vi "DES.vi"(8 "error in":errorcluster, 9 "keyStr":string="luxshare", 10 "sourceData":string="Figoba", 11 "操作":enum16{"DES_Encrypt", "DES_Decrypt"}(ring)) -> (0 "error out":errorcluster, 3 "加密后字符串":string)   [LabVIEW 2011]
uses:
  Data/DES_string.dll
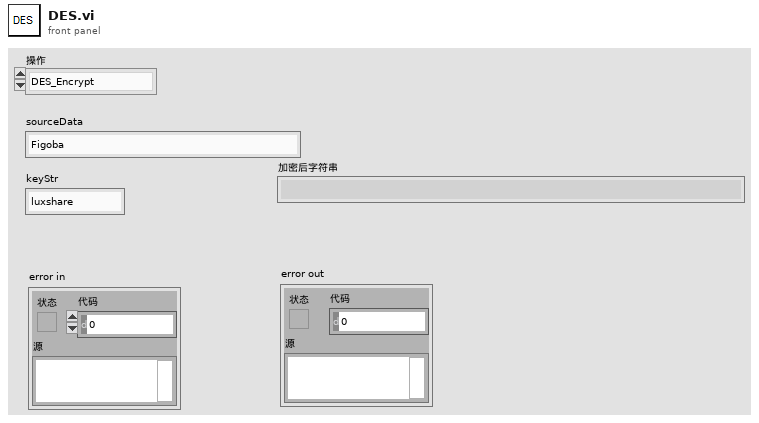
[diagram p1: front panel]
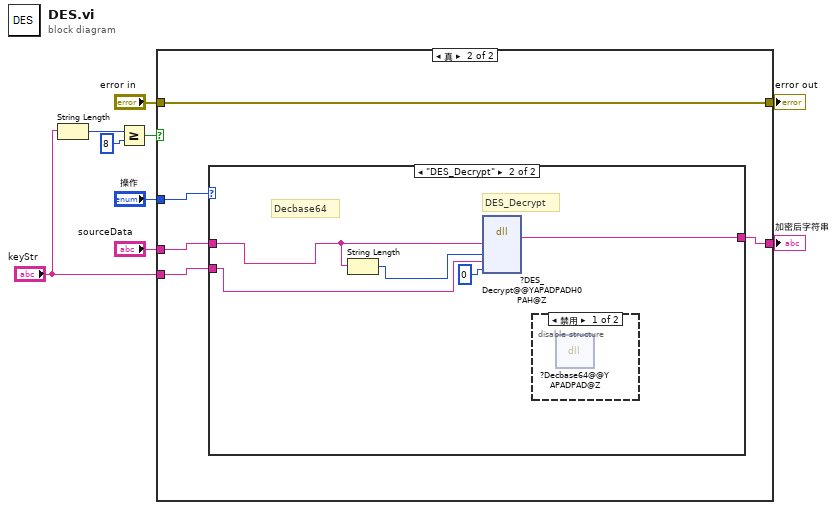
[diagram p0: block diagram]
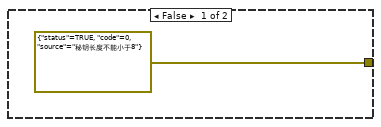
[diagram p2: hidden frame]
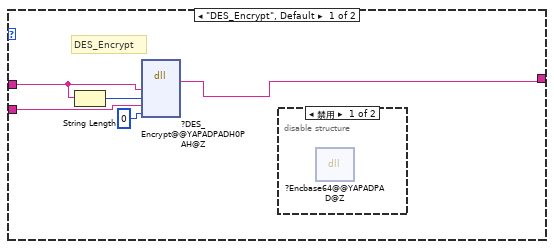
[diagram p3: hidden frame]
diagram:
  n1 = String Length(string="keyStr") -> (length=w9:i32)
  n2 = Greater Or Equal?(x=w9, y=8) -> (x >= y?=w7:bool)
  n3 = case shown="真" w7 {
    tunnel: "sourceData" -> [_ w15]
    tunnel: "操作" -> [_ w14]
    tunnel: [_ w13] -> w3
    tunnel: "keyStr" -> [_ w12]
    tunnel: [errorcluster {"status"=TRUE, "code"=0, "source"="秘钥长度不能小于8"} ("error constant") w11] -> w2
    tunnel: "error in" -> [_ w11]
    frame False {
    }
    frame True {
      n4 = case shown="\"DES_Decrypt\"" w14 {
        tunnel: w15 -> [w17 w22]
        tunnel: w12 -> [w18 w24]
        tunnel: [w16 w23] -> w13
        frame "DES_Encrypt", Default {
          # "DES_Encrypt"
          n5 = String Length(string=w17) -> (length=w20:i32)
          n6 = dll-call lib="PTH1]abs D高频房软件-2. HPTS_VNA_Rev2.7.1.3-0327最新源码备份DataDES_string.dll" fn="?DES_Encrypt@@YAPADPADH0PAH@Z"("sourceData"=w17, "sourceSize"=w20, "keyStr"=w18, "resultSize"=0) -> ("返回类型"=w16:string)  [unwired: 7 in, 2 out]
          n7 = disable-structure shown="禁用" {
            frame Disabled {
              n8 = dll-call lib="PTH1]abs D高频房软件-2. HPTS_VNA_Rev2.7.1.3-0327最新源码备份DataDES_string.dll" fn="?Encbase64@@YAPADPAD@Z"() -> ()  [unwired: 6 in, 2 out]
            }
            frame Enabled {
            }
          }
        }
        frame "DES_Decrypt" {
          # "Decbase64"
          # "DES_Decrypt"
          n9 = String Length(string=w22) -> (length=w21:i32)
          n10 = dll-call lib="PTH1]abs D高频房软件-2. HPTS_VNA_Rev2.7.1.3-0327最新源码备份DataDES_string.dll" fn="?DES_Decrypt@@YAPADPADH0PAH@Z"("sourceData"=w22, "sourceSize"=w21, "keyStr"=w24, "resultSize"=0) -> ("返回类型"=w23:string)  [unwired: 7 in, 2 out]
          n11 = disable-structure shown="禁用" {
            frame Disabled {
              n12 = dll-call lib="PTH1]abs D高频房软件-2. HPTS_VNA_Rev2.7.1.3-0327最新源码备份DataDES_string.dll" fn="?Decbase64@@YAPADPAD@Z"() -> ()  [unwired: 6 in, 2 out]
            }
            frame Enabled {
            }
          }
        }
      }
    }
  }
  "加密后字符串" <- w3
  "error out" <- w2
